vi "10-Tap 8-Bit Camera with DRAM(FPGA).vi"() -> ()   [LabVIEW 2014]
doc: "This is the FPGA VI for the 10-Tap 8-Bit Camera with DRAM example. This example demonstrates how to acquire images from a 10-tap, 8-bit, extended configuration, Camera Link camera and transfer the images to the host. This example supports area scan and line scan cameras for both continuous and finite acquisitions.\n\nThis example also demonstrates the use of DRAM as a frame buffer for very high speed acquisitions. Data packing and flow-control are also employed to maximize use of the available DRAM and FIFOs in terms of both memory space and performance.\n\nAdditionally, the example demonstrates the serial server, which allows third-party camera configuration utilities to communicate with the camera using the Camera Link serial interface while this VI is running."
uses:
  Common/CL Signal Mapping.ctl
  Common/CL Configuration.ctl
  <vilib>/Platform/TimedLoop/XDataNode/timing_clust.ctl
  <vilib>/Platform/TimedLoop/XDataNode/nitl_modes.ctl
  <vilib>/Platform/TimedLoop/XDataNode/wakeup.ctl
  <vilib>/rvi/Emulation/niFpgaGetClockAttributes.vi
  <vilib>/rvi/Emulation/niFpgaSctlEmulationGetInTimedLoop.vi
  <vilib>/rvi/Emulation/niFpgaEmulationReportErrorSimple.vi
  <vilib>/rvi/Emulation/niFpgaProcessEmulError.vi
  <vilib>/rvi/Emulation/niFpgaCriticalErrorInLSC.vi
  <vilib>/rvi/eio/common/nirviEmuTemplateMethod_errors.vi
  Common/CL Data to Pixels/10 Tap 8-Bit.vi
  <vilib>/rvi/Emulation/niFpgaEmulationIsFPGAContextNoSignature.vi
  <vilib>/rvi/FIFO/Fifo_Resource/nirvififoEmulationSetSize.vi
  <vilib>/rvi/DataTransferAndStorage/Container/Common/niFpgaContainerGetUniqueNameForEmu.vi
  <vilib>/rvi/FIFO/Fifo_Resource/nirviFifoEmulationQueueMgr.vi
  <instcachedir>/0/nirviFifoEmulationQueueMgr_E5CAEC123FF24DC58D834DCA3CDAA9B5.lvgen/nirviFifoEmulationQueueMgr_E5CAEC123FF24DC58D834DCA3CDAA9B5_001.vi
  <instcachedir>/0/nirviFifoEmulationQueueMgr_E5CAEC123FF24DC58D834DCA3CDAA9B5.lvgen/nirviFifoEmulationQueueMgr_E5CAEC123FF24DC58D834DCA3CDAA9B5_000.vi
  <vilib>/rvi/errors/niFpgaSetErrorForExecOnDevCompSimple.vi
  <vilib>/rvi/eio/common/nirviEmuReportErrorAndStop.vi
  <vilib>/rvi/FIFO/Fifo_Resource/nirvififoEmulationCreateLock.vi
  <vilib>/rvi/FIFO/Fifo_Resource/nirvififoEmulationObtainLock.vi
  <vilib>/rvi/FIFO/Fifo_Resource/nirvififoEmulationReleaseLock.vi
  <vilib>/rvi/occurrence/nirviWaitOnOccurrenceBase.vi
  <vilib>/rvi/errors/nirviReportUnexpectedCaseInternalError.vi
  <vilib>/rvi/errors/nirviReportUnexpectedCaseInternalError (U32).vi
  <vilib>/rvi/interface/RandomDataEmulation/niFpgaRandomDataHandleErrors.vi
  <vilib>/rvi/FIFO/Fifo_Resource/nirvififoEmulationDetermineInputValidOut.vi
  <vilib>/eio/EIONode/EIONode.xnode
  <vilib>/Platform/TimedLoop/XDataNode/XDataNode.xnode
  <vilib>/rvi/DataTransferAndStorage/Container/XNode/niFpgaContainer.xnode
  <vilib>/rvi/FIFO/Fifo_Resource/nirvififoEmulationGetNumberOfElementsToRead.vi
  <vilib>/rvi/FIFO/Fifo_Resource/nirvififoEmulationRead.vi
  <vilib>/rvi/interface/RandomDataEmulation/nirviRandomDataFpgaReadWriteTemplate.vi
  <vilib>/rvi/FIFO/Fifo_Resource/nirvififoEmulationWrite.vi
  <vilib>/Platform/TimedLoop/XDataNode/XDNodeRunTimeDep.lvlib
panel:
  in  "Threshold":u8
  in  "CL Config.Configuration":T1=enum."Full"
  in  "CL Config.Signal Mapping":T2=enum."Basler 10-tap"
  in  "CL Config.Line Scan":bool
  in  "CL Config.DVAL Active High":bool=TRUE
  in  "CL Config.LVAL Active High":bool=TRUE
  in  "CL Config.FVAL Active High":bool=TRUE
  in  "CL Config.Spare Active High":bool=TRUE
  in  "Acq Control.Line Scan Height":u32
  in  "Acq Control.Frames To Acq":u32
  in  "Acq Control.Acquire":bool
  in  "Acq Control.Cancel Acq":bool
  in  "Acq Control.Ignore DVAL":bool
  in  "Acq Control.Initialize":bool
  out "Acq Status.Acq In Progress":bool
  out "Acq Status.Clocks Per Line":u32
  out "Acq Status.Frames Acq'd":u32
  out "Acq Status.Lines Per Frame":u32
  out "Acq Status.DMA Write Timeout":bool
  out "Acq Status.Initialized":bool
  in  "UART.Baud Rate":u8
  in  "UART.Transmit":bool
  in  "UART.Tx Data":u8[](array[numeric])=[0, 0, 0, 0, 0, 0, 0, 0, 0, 0] format="%02x"
  in  "UART.Set Baud Rate":bool
  in  "UART.Byte Mode":bool=TRUE
  out "UART.Rx Ready":bool
  out "UART.Break Indicator":bool
  out "UART.Framing Error":bool
  out "UART.Overrun Error":bool
  out "UART.Tx Ready":bool
  out "UART.Rx Data":u8 format="%02x"
  in  "UART.Receive":bool
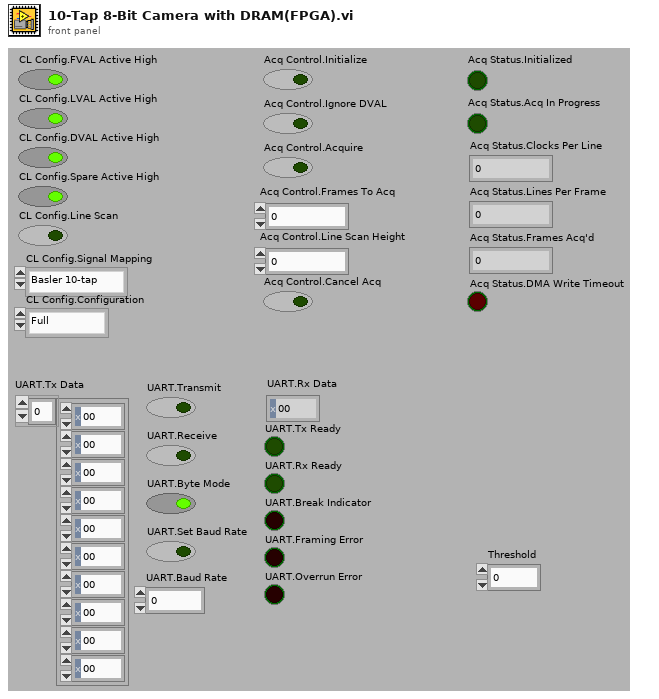
[diagram p1: front panel]
types:
  T1 = typedef "CL Configuration.ctl" = enum8{"Base", "Medium", "Full"}
  T2 = typedef "CL Signal Mapping.ctl" = enum8{"Standard", "Basler 10-tap", "Vosskühler 10-tap"}
  T3 = typedef "XDNodeRunTimeDep.lvlib/timing_clust.ctl" = cluster{"Expected End [f-1]":u64, "Actual End [f-1]":u64, "Finished Late? [f-1]":bool, "Expected End [i-1]":u64, "Actual End [i-1]":u64, "Finished Late? [i-1]":bool, "Expected Start [i]":u64, "Actual Start [i]":u64, "Expected Start [f]":u64, "Actual Start [f]":u64, "Source Name":string, "Structure Name":string, "Period":i64, "Deadline":i64, "Offset":i64, "Start":i64, "Priority":i32, "Timeout":i32, "Mode":T4, "Wakeup Reason":T5, "Error":errorcluster, "Source Type":string, "Secondary Source Type":string, "Global End Time":u64, "Global Start Time":u64, "Frame Duration":u64, "Iteration Duration":u64, "Assigned CPU":i32, "I/O Scan Engine Mode":u32}
  T4 = typedef "XDNodeRunTimeDep.lvlib/nitl_modes.ctl" = enum32{"No Change", "Process missed periods, maintain original phase", "Discard missed periods, maintain original phase", "Process missed periods, ignore original phase", "Discard missed periods, ignore original phase"}
  T5 = typedef "XDNodeRunTimeDep.lvlib/wakeup.ctl" = enum32{"Normal", "Aborted", "Asynchronous wakeup", "Timing source error", "Timed loop error", "Timeout"}
  T6 = cluster{"Enables Valid":bool, "Frame Valid":bool, "Line Valid":bool, "Data Valid":bool}
  T7 = cluster{"Pixel 0":u8, "Pixel 1":u8, "Pixel 2":u8, "Pixel 3":u8, "Pixel 4":u8, "Pixel 5":u8, "Pixel 6":u8, "Pixel 7":u8, "Pixel 8":u8, "Pixel 9":u8}
  T8 = cluster{"Tx Data":u8[], "Transmit":bool, "Receive":bool, "Byte Mode":bool, "Set Baud Rate":bool, "Baud Rate":u8}
  T9 = cluster{"Rx Data":u8, "Turn Off Transmit":bool, "Turn Off Receive":bool, "Turn Off Set Baud Rate":bool, "Tx Ready":bool, "Rx Ready":bool, "Break Indicator":bool, "Framing Error":bool, "Overrun Error":bool}
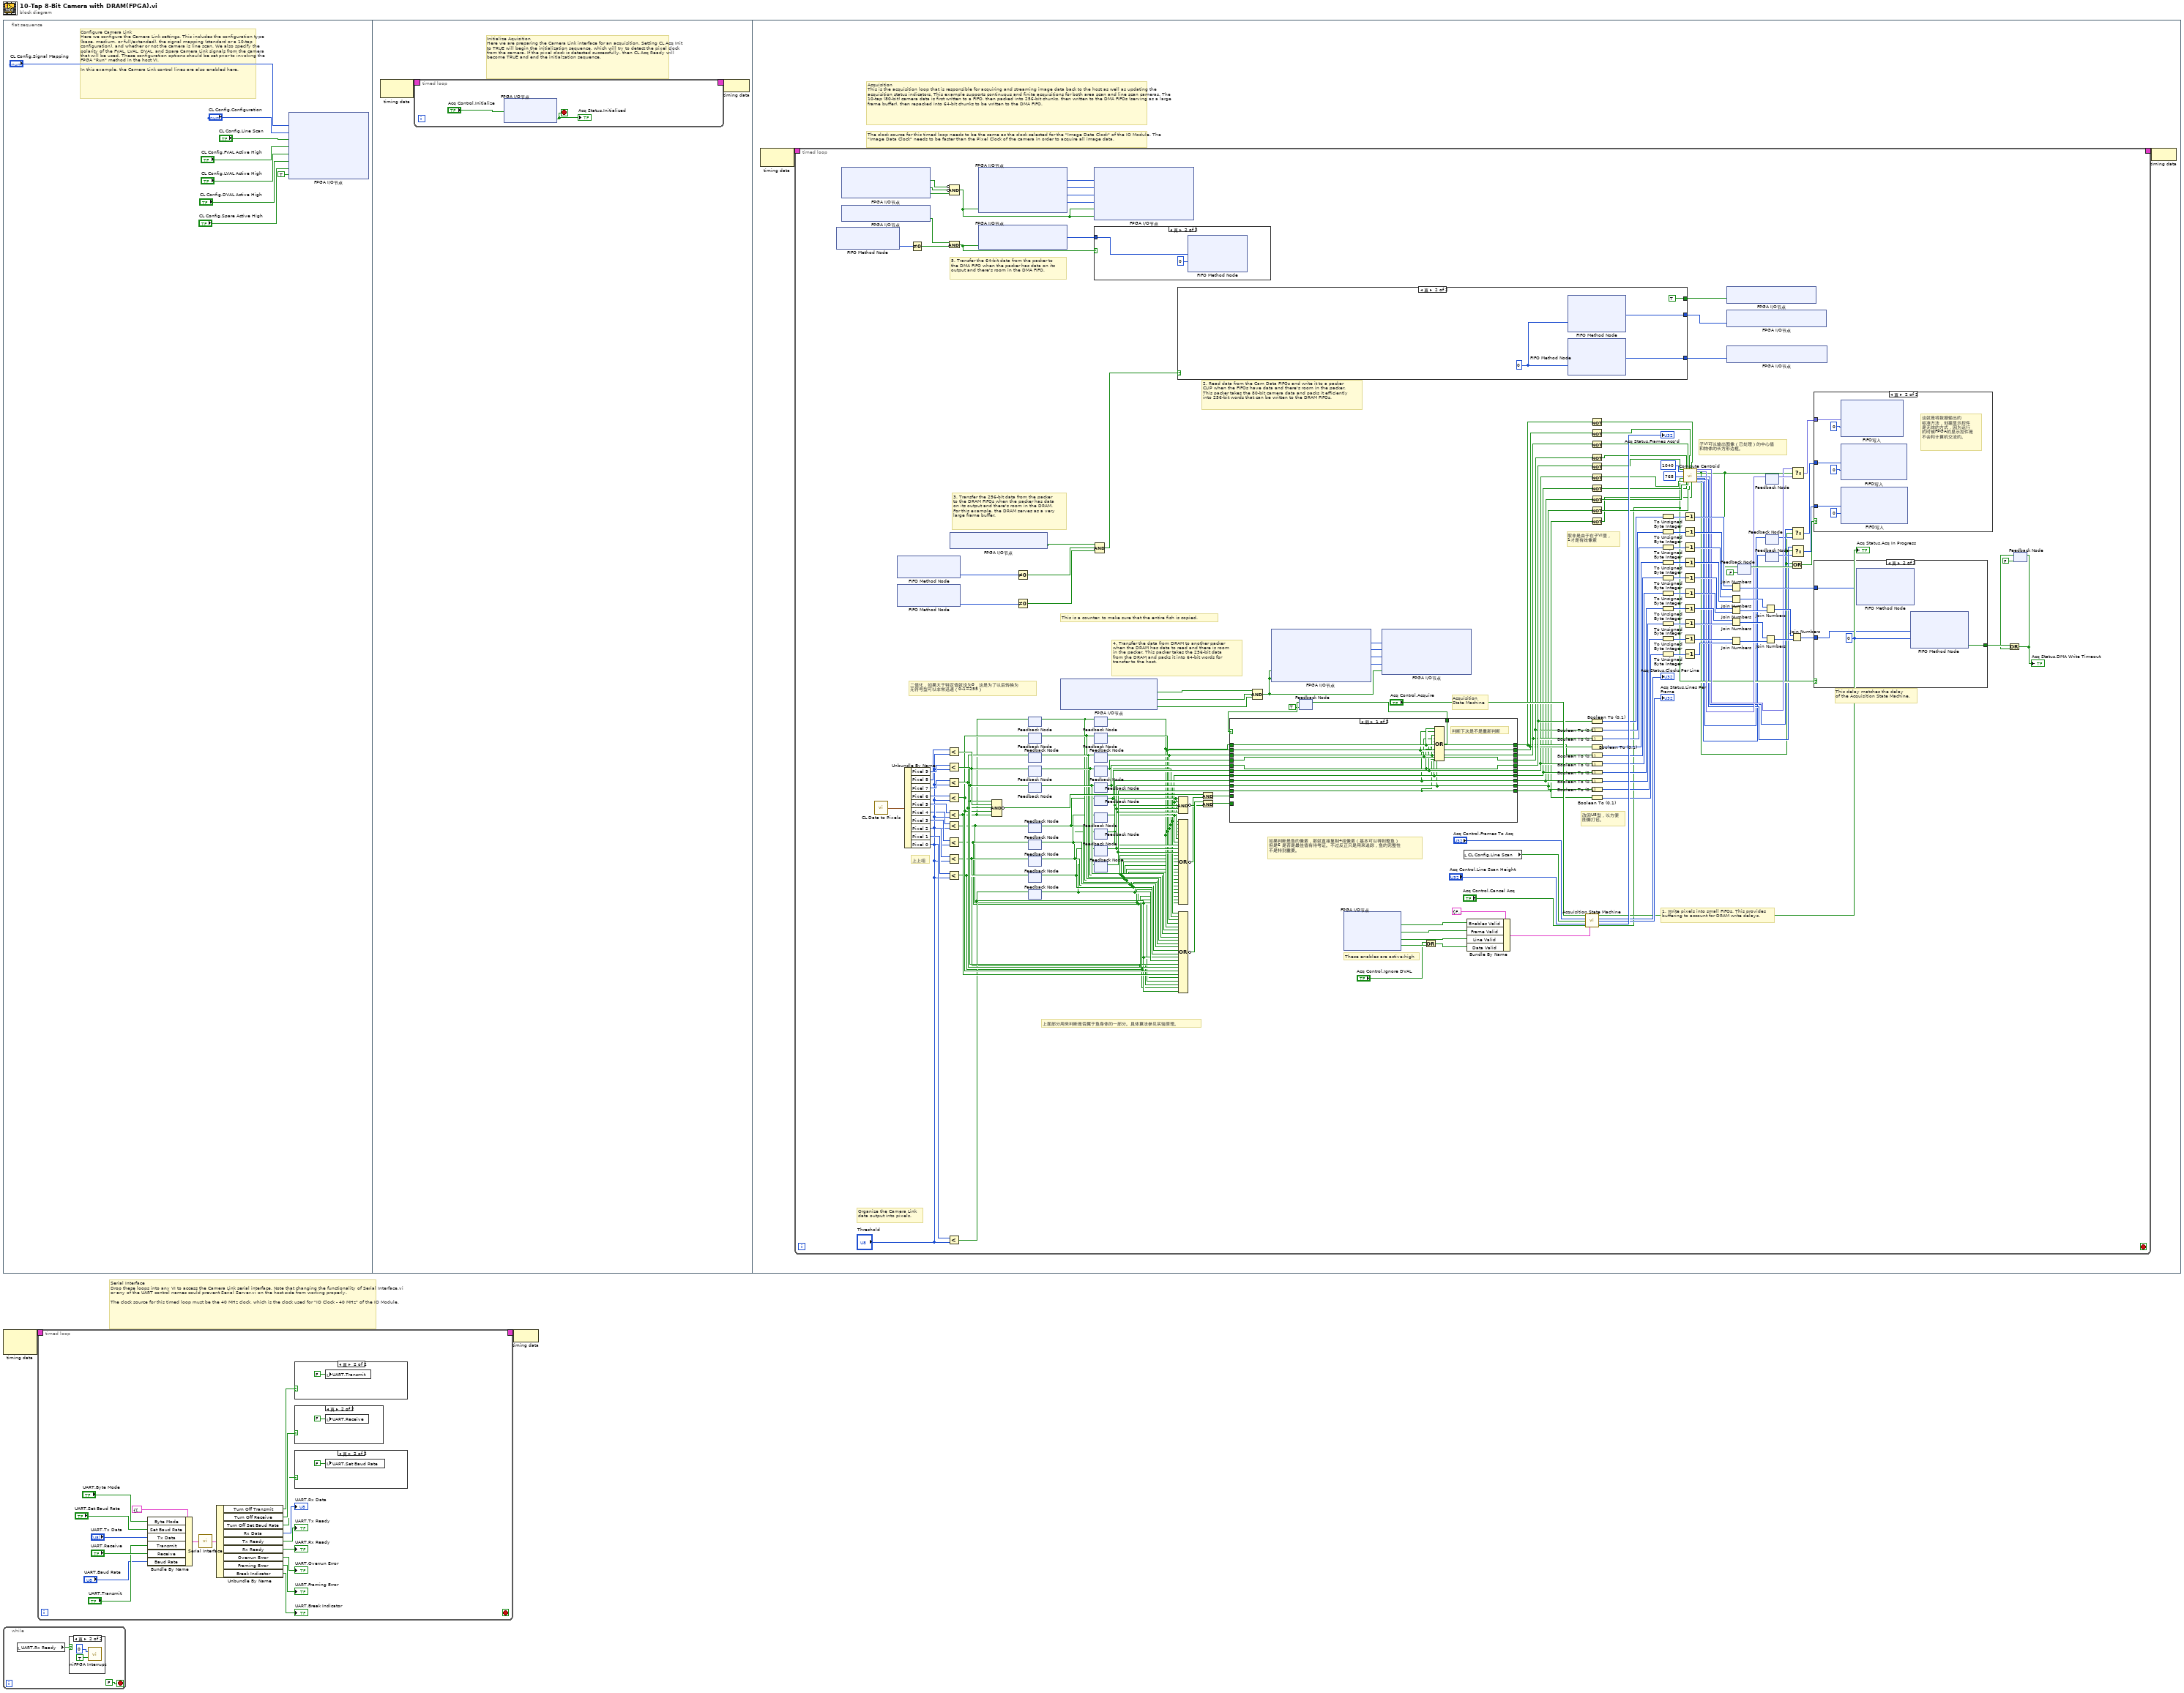
[diagram p0: block diagram]
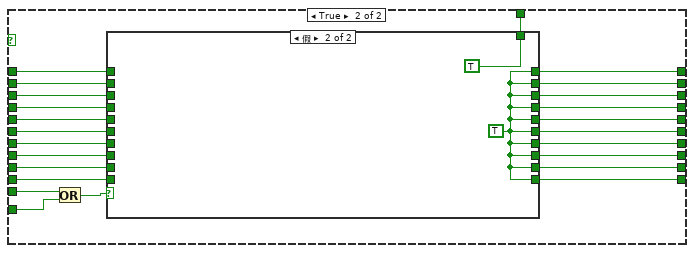
[diagram p7: hidden frame]
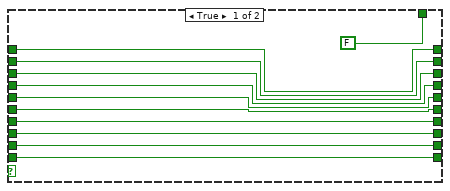
[diagram p8: hidden frame]
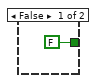
[diagram p11: hidden frame]
diagram:
  # "Serial Interface\nDrop these loops into any VI to access the Camera Link serial interface. Note that changing the functionality of Serial Interface.vi or any of the UART control names could prevent Serial Server.vi on the host side from working properly.\n\nThe clock source for this timed loop must be the 40 MHz clock, which is the clock used for \"IO Clock - 40 MHz\" of the IO Module."
  n1 = flat-sequence {
    frame #0 {
      # "Configure Camera Link\nHere we configure the Camera Link settings. This includes the configuration type (base, medium, or full/extended), the signal mapping (standard or a 10-tap configuration), and whether or not the camera is line scan. We also specify the polarity of the FVAL, LVAL, DVAL, and Spare Camera Link signals from the camera that will be used. These configuration options should be set prior to invoking the FPGA \"Run\" method in the host VI.\n\nIn this example, the Camera Link control lines are also enabled here."
      n2 = xnode "FPGA I/O节点"("CL Set Signal Mapping"="CL Config.Signal Mapping", "CL Set Configuration"="CL Config.Configuration", "CL Set Line Scan"="CL Config.Line Scan", "CL Set FVAL Active High"="CL Config.FVAL Active High", "CL Set LVAL Active High"="CL Config.LVAL Active High", "CL Set DVAL Active High"="CL Config.DVAL Active High", "CL Set Spare Active High"="CL Config.Spare Active High", "CL Control Enable"=TRUE ("IO Module\\CL Control Enable")) -> ()  [unwired: 8 in, 8 out]
    }
    frame #1 {
      # "Initialize Aquisition\nHere we are preparing the Camera Link interface for an acquisition. Setting CL Acq Init to TRUE will begin the initialization sequence, which will try to detect the pixel clock from the camera. If the pixel clock is detected successfully, then CL Acq Ready will become TRUE and end the initialzation sequence."
      n3 = node-c288() -> (w12:T3)  [unwired: 1 out]
      n4 = timed-loop {
        timing: w12 -> [_]
        timing-out: [_] -> w11
        stop <- w13 stop-if-true
        n5 = xnode "FPGA I/O节点"("CL Acq Init"="Acq Control.Initialize") -> ("CL Acq Ready"=w13:bool)  [unwired: 2 in, 2 out]
        "Acq Status.Initialized" <- w13
      }
      n6 = node-c288(w11) -> ()
    }
    frame #2 {
      # "The clock source for this timed loop needs to be the same as the clock selected for the \"Image Data Clock\" of the IO Module. The \"Image Data Clock\" needs to be faster than the Pixel Clock of the camera in order to acquire all image data."
      # "Acquisition\nThis is the acquisition loop that is responsible for acquiring and streaming image data back to the host as well as updating the acquisition status indicators. This example supports continuous and finite acquisitions for both area scan and line scan cameras. The 10-tap (80-bit) camera data is first written to a FIFO, then packed into 256-bit chunks, then written to the DMA FIFOs (serving as a large frame buffer), then repacked into 64-bit chunks to be written to the DMA FIFO."
      n7 = node-c288() -> (w20:T3)  [unwired: 1 in]
      n8 = timed-loop {
        timing: w20 -> [_]
        timing-out: [_] -> w19
        stop <- _ stop-if-true
        # "子VI可以输出图像（已处理）的中心值\n和物体的长方形边框。"
        # "取非是由于在子VI里，\n1才是有效像素"
        # "改回U8型，以方便\n图像打包。"
        # "如果判断是鱼的像素，那就直接复制4组像素（基本可以得到整鱼）\n但是6 是否是最佳值有待考证。不过反正只是用来追踪，鱼的完整性\n不是特别重要。"
        # "上面部分用来判断是否属于鱼身体的一部分。具体算法参见实验原理。"
        # "二值化，如果大于特定值就设为0，这是为了以后转换为\n无符号型可以非常迅速（0-1=255）"
        # "上上组"
        # "This is a counter, to make sure that the entire fish is copied."
        # "3. Transfer the 256-bit data from the packer\nto the DRAM FIFOs when the packer has data\non its output and there's room in the DRAM.\nFor this example, the DRAM serves as a very\nlarge frame buffer."
        # "5. Transfer the 64-bit data from the packer to\nthe DMA FIFO when the packer has data on its\noutput and there's room in the DMA FIFO."
        # "4. Transfer the data from DRAM to another packer\nwhen the DRAM has data to read and there is room\nin the packer. This packer takes the 256-bit data\nfrom the DRAM and packs it into 64-bit words for\ntransfer to the host."
        # "2. Read data from the Cam Data FIFOs and write it to a packer\nCLIP when the FIFOs have data and there's room in the packer.\nThis packer takes the 80-bit camera data and packs it efficiently\ninto 256-bit words that can be written to the DRAM FIFOs."
        # "1. Write pixels into small FIFOs. This provides\nbuffering to account for DRAM write delays."
        # "Organize the Camera Link\ndata output into pixels."
        # "These enables are active-high"
        # "This delay matches the delay\nof the Acquisition State Machine."
        # "Acquisition\nState Machine"
        n9 = xnode ("FIFO Method Node")() -> ("待写入元素数量"=w152:u32)  [unwired: 1 in, 1 out]
        n10 = xnode "FPGA I/O节点"() -> ("DRAM Bank 1\\Full"=w146:bool, "DRAM Bank 0\\Full"=w147:bool, "Pack 80 to 256\\Output Valid"=w143:bool)  [unwired: 3 in, 3 out]
        n11 = xnode "FPGA I/O节点"() -> ("Pack 256 to 64\\Output Valid"=w154:bool)  [unwired: 1 in, 1 out]
        n12 = call-poly "CL Data to Pixels.vi"() -> ("Pixels"=w199:T7)  [unwired: 1 in]
        n13 = xnode ("FIFO Method Node")() -> ("待读取元素数量"=w170:u32)  [unwired: 1 in, 1 out]
        n14 = xnode ("FIFO Method Node")() -> ("待读取元素数量"=w169:u32)  [unwired: 1 in, 1 out]
        n15 = Unbundle By Name(w199) -> ("Pixel 9"=w141:u8, "Pixel 8"=w140:u8, "Pixel 7"=w139:u8, "Pixel 6"=w138:u8, "Pixel 5"=w137:u8, "Pixel 4"=w119:u8, "Pixel 3"=w136:u8, "Pixel 2"=w135:u8, "Pixel 1"=w134:u8, "Pixel 0"=w133:u8)
        n16 = Not Equal To 0?(x=w152) -> (x != 0?=w153:bool)
        n17 = Less?(x=w140, y="Threshold") -> (x < y?=w115:bool)
        n18 = Less?(x=w141, y="Threshold") -> (x < y?=w116:bool)
        n19 = Less?(x=w139, y="Threshold") -> (x < y?=w114:bool)
        n20 = Less?(x=w138, y="Threshold") -> (x < y?=w113:bool)
        n21 = Less?(x=w137, y="Threshold") -> (x < y?=w112:bool)
        n22 = Less?(x=w119, y="Threshold") -> (x < y?=w63:bool)
        n23 = Less?(x=w136, y="Threshold") -> (x < y?=w64:bool)
        n24 = Less?(x=w135, y="Threshold") -> (x < y?=w65:bool)
        n25 = Less?(x=w134, y="Threshold") -> (x < y?=w66:bool)
        n26 = Less?(x=w133, y="Threshold") -> (x < y?=w67:bool)
        n27 = And(x=w154, y=w153) -> (x .and. y?=w142:bool)
        n28 = Compound Arithmetic op=AND(invert w146, invert w147, w143) -> (w145:bool)
        n29 = xnode "FPGA I/O节点"() -> ("Pack 80 to 256\\Ready For Write"=w166:bool)  [unwired: 1 in, 1 out]
        n30 = xnode "FPGA I/O节点"("Pack 80 to 256\\Read Enable"=w145) -> ("Pack 80 to 256\\Data Out 3"=w148:u64, "Pack 80 to 256\\Data Out 2"=w149:u64, "Pack 80 to 256\\Data Out 1"=w151:u64, "Pack 80 to 256\\Data Out 0"=w150:u64)  [unwired: 5 in, 5 out]
        n31 = xnode "FPGA I/O节点"("Pack 256 to 64\\Read Enable"=w142) -> ("Pack 256 to 64\\Data Out 64"=w159:u64)  [unwired: 2 in, 2 out]
        n32 = Compound Arithmetic op=AND(w116, w115, w114, w113, w112) -> (invert w110:bool)
        n33 = Not Equal To 0?(x=w170) -> (x != 0?=w164:bool)
        n34 = Not Equal To 0?(x=w169) -> (x != 0?=w163:bool)
        n35 = feedback #1() -> (w73:bool)  [unwired: 1 in]
        n36 = feedback-in #1(w112) -> ()
        n37 = feedback #2() -> (w74:bool)  [unwired: 1 in]
        n38 = feedback-in #2(w113) -> ()
        n39 = feedback #3() -> (w75:bool)  [unwired: 1 in]
        n40 = feedback-in #3(w114) -> ()
        n41 = feedback #4() -> (w76:bool)  [unwired: 1 in]
        n42 = feedback-in #4(w115) -> ()
        n43 = feedback-in #5(w116) -> ()
        n44 = feedback #5() -> (w77:bool)  [unwired: 1 in]
        n45 = feedback #6() -> (w72:bool)  [unwired: 1 in]
        n46 = feedback-in #6(w63) -> ()
        n47 = feedback #7() -> (w71:bool)  [unwired: 1 in]
        n48 = feedback-in #7(w64) -> ()
        n49 = feedback #8() -> (w70:bool)  [unwired: 1 in]
        n50 = feedback-in #8(w65) -> ()
        n51 = feedback #9() -> (w69:bool)  [unwired: 1 in]
        n52 = feedback-in #9(w66) -> ()
        n53 = feedback #10() -> (w68:bool)  [unwired: 1 in]
        n54 = feedback-in #10(w67) -> ()
        n55 = xnode "FPGA I/O节点"() -> ("DRAM Bank 1\\Data_Available"=w162:bool, "DRAM Bank 0\\Data_Available"=w160:bool, "Pack 256 to 64\\Ready for Write"=w161:bool)  [unwired: 3 in, 3 out]
        n56 = xnode "FPGA I/O节点"("DRAM Bank 1\\Write_Data_Upper"=w148, "DRAM Bank 1\\Write_Data_Lower"=w149, "DRAM Bank 0\\Write_Data_Upper"=w151, "DRAM Bank 0\\Write_Data_Lower"=w150, "DRAM Bank 1\\Write"=w145, "DRAM Bank 0\\Write"=w145) -> ()  [unwired: 6 in, 6 out]
        n57 = case shown="真" w142 {
          tunnel: w159 -> [_ w255]
          frame False {
          }
          frame True {
            n58 = xnode ("FIFO Method Node")("元素"=w255, "超时"=0 ("Timeout")) -> ()  [unwired: 1 in, 2 out]
          }
        }
        n59 = feedback #11() -> (w78:bool)  [unwired: 1 in]
        n60 = feedback-in #11(w73) -> ()
        n61 = feedback #12() -> (w79:bool)  [unwired: 1 in]
        n62 = feedback-in #12(w74) -> ()
        n63 = feedback #13() -> (w80:bool)  [unwired: 1 in]
        n64 = feedback-in #13(w75) -> ()
        n65 = feedback #14() -> (w81:bool)  [unwired: 1 in]
        n66 = feedback-in #14(w76) -> ()
        n67 = feedback #15() -> (w82:bool)  [unwired: 1 in]
        n68 = feedback-in #15(w77) -> ()
        n69 = feedback #16() -> (w103:bool)  [unwired: 1 in]
        n70 = feedback-in #16(w72) -> ()
        n71 = feedback #17() -> (w104:bool)  [unwired: 1 in]
        n72 = feedback-in #17(w71) -> ()
        n73 = feedback #18() -> (w105:bool)  [unwired: 1 in]
        n74 = feedback-in #18(w70) -> ()
        n75 = feedback #19() -> (w106:bool)  [unwired: 1 in]
        n76 = feedback-in #19(w69) -> ()
        n77 = feedback #20() -> (w107:bool)  [unwired: 1 in]
        n78 = feedback-in #20(w68) -> ()
        n79 = Compound Arithmetic op=AND(w166, w164, w163) -> (w165:bool)
        n80 = case shown="真" w165 {
          tunnel: [_ w259] -> w171
          tunnel: [_ w258] -> w167
          tunnel: [_ TRUE] -> w168
          frame False {
          }
          frame True {
            w257 = 0 ("Timeout")
            n81 = xnode ("FIFO Method Node")("超时"=w257) -> ("元素"=w258:u64)  [unwired: 1 in, 2 out]
            n82 = xnode ("FIFO Method Node")("超时"=w257) -> ("元素"=w259:u16)  [unwired: 1 in, 2 out]
          }
        }
        n83 = Compound Arithmetic op=AND(w103, w104, w105, w106, w107) -> (invert w117:bool)
        n84 = Compound Arithmetic op=OR(w82, w81, w80, w79, w78, w103, w104, w105, w106, w107, w77, w76, w75, w74, w73, w72, w71, w70, w69, w68, w63, w64, w65, w66, w67) -> (invert w111:bool)
        n85 = Compound Arithmetic op=OR(w82, w81, w80, w79, w78, w77, w76, w75, w74, w73, w71, w70, w69, w67, w68, w116, w114, w113, w112, w63, w64, w65, w66, w67) -> (invert w118:bool)
        n86 = And(x=w110, y=w111) -> (x .and. y?=w109:bool)
        n87 = And(x=w118, y=w117) -> (x .and. y?=w108:bool)
        n88 = Compound Arithmetic op=AND(w162, w160, w161) -> (w144:bool)
        n89 = xnode "FPGA I/O节点"("DRAM Bank 1\\Read"=w144, "DRAM Bank 0\\Read"=w144) -> ("DRAM Bank 1\\Read_Data_Upper"=w158:u64, "DRAM Bank 1\\Read_Data_Lower"=w157:u64, "DRAM Bank 0\\Read_Data_Upper"=w156:u64, "DRAM Bank 0\\Read_Data_Lower"=w155:u64)  [unwired: 6 in, 6 out]
        n90 = feedback #21(TRUE) -> (w23:bool)
        n91 = case shown="假" w23 {
          tunnel: w82 -> [w212 w227]
          tunnel: w81 -> [w213 w226]
          tunnel: w80 -> [w214 w225]
          tunnel: w79 -> [w215 w224]
          tunnel: w78 -> [w216 w223]
          tunnel: w103 -> [w211 w222]
          tunnel: w104 -> [w210 w221]
          tunnel: w105 -> [w209 w220]
          tunnel: w106 -> [w208 w219]
          tunnel: w107 -> [w207 w218]
          tunnel: [w212 w240] -> w53
          tunnel: [w213 w239] -> w52
          tunnel: [w214 w238] -> w51
          tunnel: [w215 w237] -> w50
          tunnel: [w216 w236] -> w49
          tunnel: [w211 w235] -> w48
          tunnel: [w210 w234] -> w47
          tunnel: [w209 w233] -> w46
          tunnel: [w208 w232] -> w45
          tunnel: [w207 w231] -> w44
          tunnel: w109 -> [_ w229]
          tunnel: w108 -> [_ w228]
          tunnel: [w206 w217] -> w22
          frame False {
            # "判断下次是不是重新判断"
            n92 = Compound Arithmetic op=OR(w216, w215, w214, w213, w212, w211, w210, w209, w208, w207) -> (w206:bool)
          }
          frame True {
            n93 = Or(x=w229, y=w228) -> (x .or. y?=w230:bool)
            n94 = case shown="假" w230 {
              tunnel: [w251 w253] -> w240
              tunnel: [w250 w253] -> w239
              tunnel: [w249 w253] -> w238
              tunnel: [w242 w253] -> w231
              tunnel: [w248 w253] -> w237
              tunnel: [w247 w253] -> w236
              tunnel: [w246 w253] -> w235
              tunnel: [w245 w253] -> w234
              tunnel: [w244 w253] -> w233
              tunnel: [w243 w253] -> w232
              tunnel: w227 -> [w251 _]
              tunnel: w226 -> [w250 _]
              tunnel: w225 -> [w249 _]
              tunnel: w224 -> [w248 _]
              tunnel: w223 -> [w247 _]
              tunnel: w222 -> [w246 _]
              tunnel: w221 -> [w245 _]
              tunnel: w220 -> [w244 _]
              tunnel: w219 -> [w243 _]
              tunnel: w218 -> [w242 _]
              tunnel: [FALSE TRUE] -> w217
              frame True {
              }
              frame False {
                w253 = TRUE
              }
            }
          }
        }
        n95 = feedback-in #21(w22) -> ()
        n96 = xnode "FPGA I/O节点"() -> ("CL Output Valid"=w187:bool, "CL Frame Valid"=w186:bool, "CL Line Valid"=w185:bool, "CL Data Valid"=w182:bool)  [unwired: 4 in, 4 out]
        n97 = xnode "FPGA I/O节点"("Pack 256 to 64\\Data In 3"=w158, "Pack 256 to 64\\Data In 2"=w157, "Pack 256 to 64\\Data In 1"=w156, "Pack 256 to 64\\Data In 0"=w155, "Pack 256 to 64\\Write Enable"=w144) -> ()  [unwired: 5 in, 5 out]
        n98 = Or(x="Acq Control.Ignore DVAL", y=w182) -> (x .or. y?=w181:bool)
        n99 = local read "CL Config.Line Scan"() -> (w179:bool)
        n100 = Bundle By Name(cluster=T6 {"Enables Valid"=FALSE, "Frame Valid"=FALSE, "Line Valid"=FALSE, "Data Valid"=FALSE} ("Enables"), "Enables Valid"=w187, "Frame Valid"=w186, "Line Valid"=w185, "Data Valid"=w181) -> (w184:T6)
        n101 = call "Acquisition State Machine.vi"("Acquire"="Acq Control.Acquire", "Frames to Acquire"="Acq Control.Frames To Acq", "Line Scan"=w179, "Line Scan Height"="Acq Control.Line Scan Height", "Cancel Acq"="Acq Control.Cancel Acq", "Enables"=w184) -> ("Acq In Progress"=→"Acq Status.Acq In Progress":bool, "Num Clocks Per Line"=→"Acq Status.Clocks Per Line":u32, "Num Lines Per Frame"=→"Acq Status.Lines Per Frame":u32, "Num Frames Acq'd"=→"Acq Status.Frames Acq'd":u32, "Capture Cycle"=w35:bool)  [unwired: 4 in, 1 out]
        n102 = Not(x=w49) -> (.not. x?=w43:bool)
        n103 = Not(x=w50) -> (.not. x?=w40:bool)
        n104 = Not(x=w51) -> (.not. x?=w33:bool)
        n105 = Not(x=w52) -> (.not. x?=w41:bool)
        n106 = Not(x=w53) -> (.not. x?=w42:bool)
        n107 = Not(x=w48) -> (.not. x?=w38:bool)
        n108 = Not(x=w47) -> (.not. x?=w37:bool)
        n109 = Not(x=w46) -> (.not. x?=w39:bool)
        n110 = Not(x=w45) -> (.not. x?=w36:bool)
        n111 = Not(x=w44) -> (.not. x?=w34:bool)
        n112 = Boolean To (0,1)(Boolean=w53) -> (0, 1=w102:i16)
        n113 = Boolean To (0,1)(Boolean=w52) -> (0, 1=w100:i16)
        n114 = Boolean To (0,1)(Boolean=w51) -> (0, 1=w98:i16)
        n115 = Boolean To (0,1)(Boolean=w50) -> (0, 1=w96:i16)
        n116 = Boolean To (0,1)(Boolean=w49) -> (0, 1=w94:i16)
        n117 = Boolean To (0,1)(Boolean=w48) -> (0, 1=w92:i16)
        n118 = Boolean To (0,1)(Boolean=w47) -> (0, 1=w90:i16)
        n119 = Boolean To (0,1)(Boolean=w46) -> (0, 1=w88:i16)
        n120 = Boolean To (0,1)(Boolean=w45) -> (0, 1=w86:i16)
        n121 = Boolean To (0,1)(Boolean=w44) -> (0, 1=w84:i16)
        n122 = To Unsigned Byte Integer(number=w102) -> (unsigned 8bit integer=w101:u8)
        n123 = To Unsigned Byte Integer(number=w100) -> (unsigned 8bit integer=w99:u8)
        n124 = To Unsigned Byte Integer(number=w98) -> (unsigned 8bit integer=w97:u8)
        n125 = To Unsigned Byte Integer(number=w96) -> (unsigned 8bit integer=w95:u8)
        n126 = To Unsigned Byte Integer(number=w94) -> (unsigned 8bit integer=w93:u8)
        n127 = To Unsigned Byte Integer(number=w92) -> (unsigned 8bit integer=w91:u8)
        n128 = To Unsigned Byte Integer(number=w90) -> (unsigned 8bit integer=w89:u8)
        n129 = To Unsigned Byte Integer(number=w88) -> (unsigned 8bit integer=w87:u8)
        n130 = To Unsigned Byte Integer(number=w86) -> (unsigned 8bit integer=w85:u8)
        n131 = To Unsigned Byte Integer(number=w84) -> (unsigned 8bit integer=w83:u8)
        n132 = Decrement(x=w101) -> (x-1=w130:u8)
        n133 = Decrement(x=w99) -> (x-1=w129:u8)
        n134 = Decrement(x=w97) -> (x-1=w128:u8)
        n135 = Decrement(x=w95) -> (x-1=w127:u8)
        n136 = Decrement(x=w93) -> (x-1=w126:u8)
        n137 = Decrement(x=w91) -> (x-1=w125:u8)
        n138 = Decrement(x=w89) -> (x-1=w124:u8)
        n139 = Decrement(x=w87) -> (x-1=w123:u8)
        n140 = Decrement(x=w85) -> (x-1=w122:u8)
        n141 = Decrement(x=w83) -> (x-1=w121:u8)
        n142 = call "Compute Centroid.vi"("Pixel0"=w42, "Image Width"=u16 1040, "Image Height"=u16 768, "Input Valid"=w35, "Pixel5"=w38, "Pixel1"=w41, "Pixel6"=w37, "Pixel2"=w33, "Pixel7"=w39, "Pixel3"=w40, "Pixel8"=w36, "Pixel4"=w43, "Pixel9"=w34) -> ("X"=w57:fxp<+,32,16>, "Y"=w56:fxp<+,32,16>, "Output valid"=w25:bool, "Ymin"=w28:u16, "Ymax"=w27:u16, "Xmin"=w32:u16, "Xmax"=w31:u16)  [unwired: 8 in]
        n143 = xnode "FPGA I/O节点"("Pack 80 to 256\\Write Enable"=w168) -> ()  [unwired: 1 in, 1 out]
        n144 = xnode "FPGA I/O节点"("Pack 80 to 256\\Data In Lower 64"=w167) -> ()  [unwired: 1 in, 1 out]
        n145 = xnode "FPGA I/O节点"("Pack 80 to 256\\Data In Upper 16"=w171) -> ()  [unwired: 1 in, 1 out]
        n146 = Join Numbers(hi=w130, lo=w129) -> ((hi.lo)=w132:u16)
        n147 = Join Numbers(hi=w128, lo=w127) -> ((hi.lo)=w176:u16)
        n148 = Join Numbers(hi=w126, lo=w125) -> ((hi.lo)=w175:u16)
        n149 = Join Numbers(hi=w124, lo=w123) -> ((hi.lo)=w174:u16)
        n150 = Join Numbers(hi=w122, lo=w121) -> ((hi.lo)=w177:u16)
        n151 = feedback #22(FALSE ("Output valid")) -> (w60:bool)
        n152 = feedback-in #22(w25) -> ()
        n153 = Join Numbers(hi=w176, lo=w175) -> ((hi.lo)=w173:u32)
        n154 = Join Numbers(hi=w174, lo=w177) -> ((hi.lo)=w172:u32)
        n155 = feedback #23() -> (w59:fxp<+,32,16>)  [unwired: 1 in]
        n156 = feedback-in #23(w56) -> ()
        n157 = feedback #24() -> (w26:u16)  [unwired: 1 in]
        n158 = feedback-in #24(w27) -> ()
        n159 = feedback #25() -> (w30:u16)  [unwired: 1 in]
        n160 = feedback-in #25(w31) -> ()
        n161 = Or(x=w25, y=w60) -> (x .or. y?=w62:bool)
        n162 = Join Numbers(hi=w173, lo=w172) -> ((hi.lo)=w131:u64)
        n163 = Select(t=w57, s=w25, f=w59) -> (s? t:f=w61:fxp<+,32,16>)
        n164 = Select(t=w28, s=w25, f=w26) -> (s? t:f=w24:u16)
        n165 = Select(t=w32, s=w25, f=w30) -> (s? t:f=w29:u16)
        n166 = case shown="真" w62 {
          tunnel: w61 -> [_ w205]
          tunnel: w29 -> [_ w203]
          tunnel: w24 -> [_ w200]
          frame False {
          }
          frame True {
            # "这就是将数据输出的\n标准方法，创建显示控件\n是无效的方式，因为运行\n的时候FPGA的显示控件是\n不会和计算机交流的。"
            n167 = xnode ("FIFO写入")("元素"=w205, "超时"=0 ("Timeout")) -> ()  [unwired: 1 in, 2 out]
            n168 = xnode "FIFO写入"("元素"=w200, "超时"=0) -> ()  [unwired: 1 in, 2 out]
            n169 = xnode ("FIFO写入")("元素"=w203, "超时"=0) -> ()  [unwired: 1 in, 2 out]
          }
        }
        n170 = case shown="真" w35 {
          tunnel: [FALSE ("Timed Out?") w263] -> w197
          tunnel: w131 -> [_ w264]
          tunnel: w132 -> [_ w262]
          frame False {
          }
          frame True {
            w261 = 0 ("Timeout")
            n171 = xnode ("FIFO Method Node")("元素"=w262, "超时"=w261) -> ()  [unwired: 1 in, 2 out]
            n172 = xnode ("FIFO Method Node")("元素"=w264, "超时"=w261) -> ("超时？"=w263:bool)  [unwired: 1 in, 1 out]
          }
        }
        n173 = feedback #26(FALSE) -> (w196:bool)
        n174 = Or(x=w197, y=w196) -> (x .or. y?=w195:bool)
        "Acq Status.DMA Write Timeout" <- w195
        n175 = feedback-in #26(w195) -> ()
      }
      n176 = node-c288(w19) -> ()
    }
  }
  n177 = node-c288() -> (w2:T3)  [unwired: 2 in]
  n178 = while {
    stop <- FALSE stop-if-true
    n179 = local read "UART.Rx Ready"() -> (w270:bool)
    n180 = case shown="真" w270 {
      frame False {
      }
      frame True {
        n181 = call <vilib>:"niFPGA Interrupt.vi"("Wait Until Cleared (F)"=TRUE ("Wait Until Cleared"), "IRQ Number (0)"=u8 0 ("IRQ Number")) -> ()  [unwired: 1 in]
      }
    }
  }
  n182 = timed-loop {
    timing: w2 -> [_]
    timing-out: [_] -> w1
    stop <- _ stop-if-true
    n183 = Bundle By Name(cluster=T8 {"Tx Data"=[0, 0, 0, 0, 0, 0, 0, 0, 0, 0], "Transmit"=FALSE, "Receive"=FALSE, "Byte Mode"=TRUE, "Set Baud Rate"=FALSE, "Baud Rate"=0} ("UART Inputs"), "Byte Mode"="UART.Byte Mode", "Set Baud Rate"="UART.Set Baud Rate", "Tx Data"="UART.Tx Data", "Transmit"="UART.Transmit", "Receive"="UART.Receive", "Baud Rate"="UART.Baud Rate") -> (w273:T8)
    n184 = call "Serial Interface.vi"("UART Inputs"=w273) -> ("UART Outputs"=w285:T9)
    n185 = Unbundle By Name(w285) -> ("Turn Off Transmit"=w278:bool, "Turn Off Receive"=w279:bool, "Turn Off Set Baud Rate"=w275:bool, "Rx Data"=→"UART.Rx Data":u8, "Tx Ready"=→"UART.Tx Ready":bool, "Rx Ready"=→"UART.Rx Ready":bool, "Overrun Error"=→"UART.Overrun Error":bool, "Framing Error"=→"UART.Framing Error":bool, "Break Indicator"=→"UART.Break Indicator":bool)
    n186 = case shown="真" w278 {
      frame False {
      }
      frame True {
        n187 = local write "UART.Transmit"(FALSE ("UART.Transmit")) -> ()
      }
    }
    n188 = case shown="真" w279 {
      frame False {
      }
      frame True {
        n189 = local write "UART.Receive"(FALSE ("UART.Receive")) -> ()
      }
    }
    n190 = case shown="真" w275 {
      frame False {
      }
      frame True {
        n191 = local write "UART.Set Baud Rate"(FALSE ("UART.Receive")) -> ()
      }
    }
  }
  n192 = node-c288(w1) -> ()
